vi "Get Component Dependencies.vi"(8 "error in (no error)":errorcluster, 10 "Target Type":T1, 11 "component paths":path[](array[path])) -> (0 "error out":errorcluster, 3 "component dependencies":T2[](array[typedef]))   [LabVIEW 2021, in "DSF System Explorer.lvlib"]
uses:
  DSF System Explorer.lvlib
  <vilib>/NI VeriStand/Custom Device API/Custom Device File Dependency.ctl
  <vilib>/NI VeriStand/Custom Device API/Path Specification.ctl
  <vilib>/NI VeriStand/Custom Device API/Path Type.ctl
  <vilib>/NI VeriStand/Custom Device API/Custom Device Supported Target.ctl
  <vilib>/NI VeriStand/Custom Device API/Custom Device Target Type.ctl
  <vilib>/NI VeriStand/Custom Device API/Custom Device API.lvlib
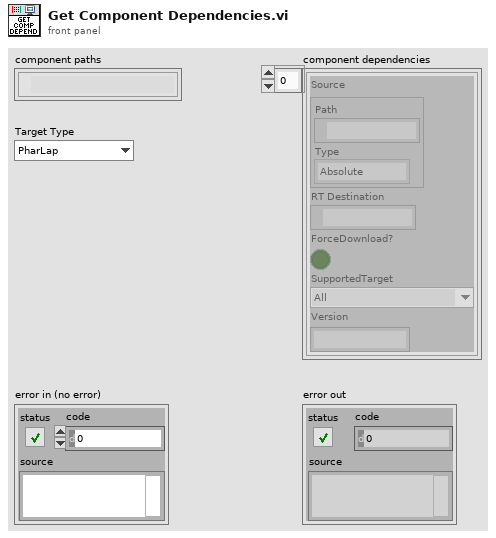
[diagram p1: front panel]
types:
  T1 = typedef "Custom Device API.lvlib/Custom Device Target Type.ctl" = enum16{"PharLap", "VxWorks", "Windows", "Linux_32_ARM", "Linux_x64"}
  T2 = typedef "Custom Device API.lvlib/Custom Device File Dependency.ctl" = cluster{"Source":T3, "RT Destination":path, "ForceDownload?":bool, "SupportedTarget":T5, "Version":string}
  T3 = typedef "Custom Device API.lvlib/Path Specification.ctl" = cluster{"Path":path, "Type":T4}
  T4 = typedef "Custom Device API.lvlib/Path Type.ctl" = enum16{"Absolute", "To Base", "To Common Data Dir", "To Application Data Dir"}
  T5 = typedef "Custom Device API.lvlib/Custom Device Supported Target.ctl" = enum16{"All", "PharLap", "VxWorks", "Windows", "Linux_32_ARM", "Linux_x64", "PharLap & Windows", "PharLap & VxWorks", "VxWorks & Windows"}
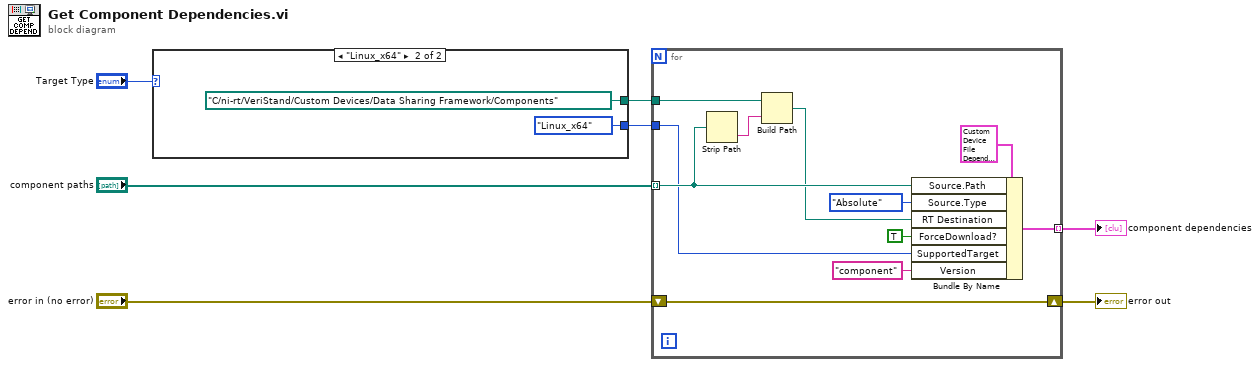
[diagram p0: block diagram]
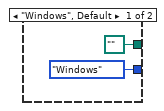
[diagram p2: hidden frame]
diagram:
  n1 = case shown="\"Linux_x64\"" "Target Type" {
    tunnel: [Custom_Device_Supported_Target."Windows" ("SupportedTarget") Custom_Device_Supported_Target."Linux_x64" ("SupportedTarget")] -> w3
    tunnel: [path "" ("RT Destination") path "C:/ni-rt/VeriStand/Custom Devices/Data Sharing Framework/Components" ("RT Destination")] -> w2
    frame "Windows", Default {
    }
    frame "Linux_x64" {
    }
  }
  n2 = for {
    tunnel: "component paths" -> [w19] mode=indexing
    shift-right: [w16] -> w6
    shift-left: "error in (no error)" -> [w16]
    tunnel: [w17] -> w5 mode=indexing
    tunnel: w3 -> [w14]
    tunnel: w2 -> [w15]
    n3 = Strip Path(path=w19) -> (name=w13:string)  [unwired: 1 out]
    n4 = Build Path(base path=w15, name or relative path=w13) -> (appended path=w18:path)
    n5 = Bundle By Name(cluster=T2 {"Source"={"Path"=path "", "Type"=enum."Absolute"}, "RT Destination"=path "", "ForceDownload?"=FALSE, "SupportedTarget"=enum."PharLap", "Version"=""} ("Dependencies"), "Source.Path"=w19, "Source.Type"=Path_Type."Absolute", "RT Destination"=w18, "ForceDownload?"=TRUE, "SupportedTarget"=w14, "Version"="component") -> (w17:T2)
  }
  "error out" <- w6
  "component dependencies" <- w5
